vi "NIIE_Line.vi"(6 "Color(black)":u32(colorbox), 8 "Error":errorcluster, 9 "End Point":cluster{"x":i16, "y":i16}, 11 "New Position":cluster{"x":i16, "y":i16}) -> (0 "Error Out":errorcluster, 3 "New Picture Out":picture)   [LabVIEW 2021]
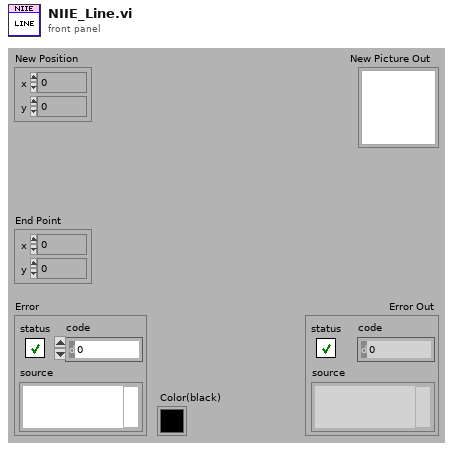
[diagram p1: front panel]
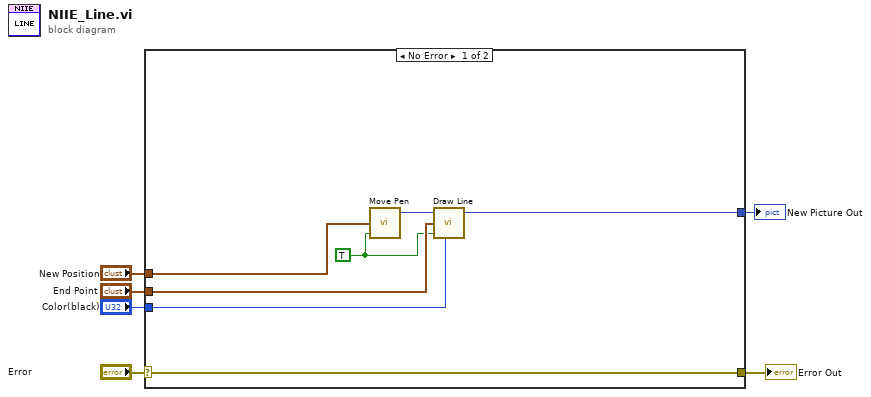
[diagram p0: block diagram]
diagram:
  n1 = case shown="No Error" "Error" {
    selector: "Error" -> [w13 w14]
    tunnel: [w13 w14] -> w5
    tunnel: "End Point" -> [w11 _]
    tunnel: "New Position" -> [w10 _]
    tunnel: "Color(black)" -> [w8 _]
    tunnel: [w7 _] -> w1
    frame No Error {
      w9 = TRUE ("absolute coordinates?(T)")
      n2 = call <vilib>:"Move Pen.vi"("absolute coordinates?(T)"=w9, "new position"=w10) -> ("new picture"=w12:picture)  [unwired: 1 in, 2 out]
      n3 = call <vilib>:"Draw Line.vi"("picture"=w12, "end point"=w11, "absolute coordinates?(T)"=w9, "color(black)"=w8) -> ("new picture"=w7:picture)  [unwired: 1 in, 4 out]
    }
    frame Error {
    }
  }
  "Error Out" <- w5
  "New Picture Out" <- w1
